vi "Queues vs Local Variables.vi"() -> ()   [LabVIEW 2011]
panel:
  in  "루프 속도(ms)":u16(ring)=50 caption="루프 속도" items=["생산자 루프와 같음"=50, "최대 속도"=0, "생산자의 2x"=25, "생산자의 1/2"=100, "생산자의 1/20"=1000]
  out "놓친 포인트 개수":i32
  in  "루프 속도(ms)":u16(ring)=50 caption="루프 속도" items=["생산자 루프와 같음"=50, "최대 속도"=0, "생산자의 2x"=25, "생산자의 1/2"=100, "생산자의 1/20"=1000]
  out "큐의 원소 개수":i32(slide) scale=0.0..1000.0
  out "생산자 루프가 \n생성한 포인트 개수":i32 caption="생산자 루프가 생성한 포인트 개수"
  in  "정지":bool
  out "로컬 변수 소비자 루프":dbl(graph) caption="사인"
  out "큐 소비자 루프":dbl(graph)=-9.510565162951542 caption="사인"
  out "생산자 루프":dbl(graph) caption="사인"
  # "생산자 루프"
  # "루프 시간 = 50 ms"
  # "로컬 변수 소비자 루프"
  # "큐 소비자 루프"
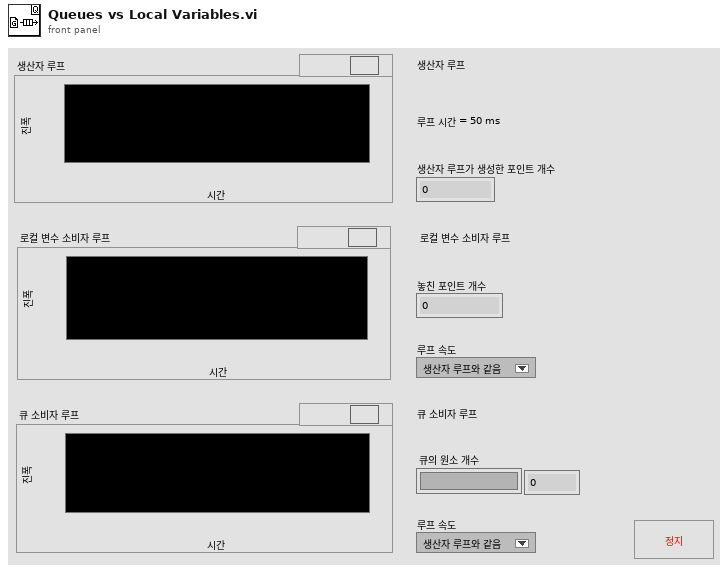
[diagram p1: front panel]
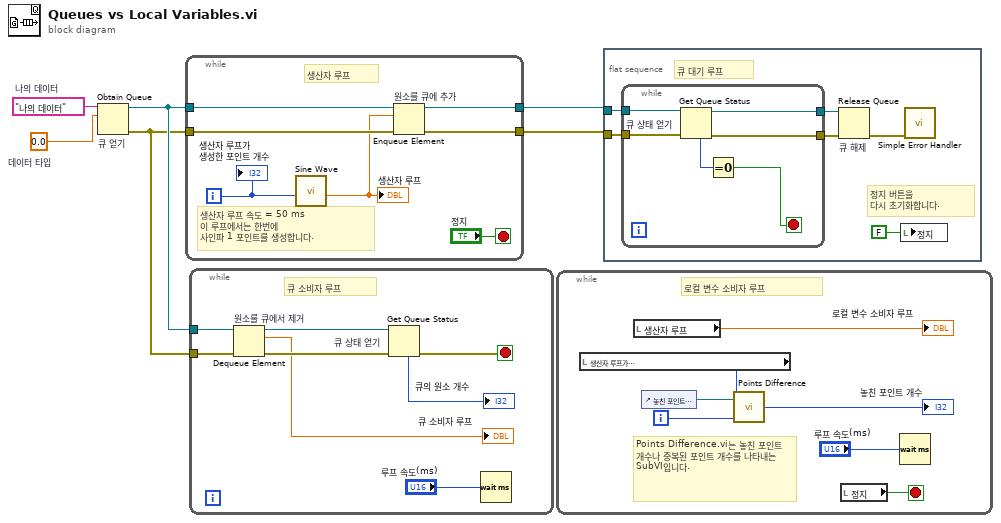
[diagram p0: block diagram]
diagram:
  w5 = "나의 데이터"  # 나의 데이터
  w6 = 0.0  # 데이터 타입
  n1 = Obtain Queue "큐 얻기"(name (unnamed)=w5, element data type=w6) -> (queue out=w4:refnum<queue>, error out=w2:errorcluster)  [unwired: 3 in, 1 out]
  n2 = while {
    tunnel: w4 -> [w11]
    tunnel: w2 -> [w10]
    tunnel: [w8] -> w1
    tunnel: [w7] -> w3
    i -> [w12]
    stop <- "정지" stop-if-true
    # "생산자 루프"
    # "생산자 루프 속도 = 50 ms\n이 루프에서는 한번에 \n사인파 1 포인트를 생성합니다."
    n3 = call "Sine Wave.vi"("숫자형"=w12) -> ("사인파"=w9:dbl)  [unwired: 6 out]
    "생산자 루프" <- w9
    n4 = Enqueue Element "원소를 큐에 추가"(queue=w11, element=w9, error in (no error)=w10) -> (queue out=w7:refnum<queue>, error out=w8:errorcluster)  [unwired: 2 out]
    "생산자 루프가 \n생성한 포인트 개수" <- w12
  }
  n5 = while {
    tunnel: w4 -> [w18]
    tunnel: w2 -> [w17]
    stop <- w15 stop-if-true
    # "큐 소비자 루프"
    n6 = Dequeue Element "원소를 큐에서 제거"(queue=w18, error in (no error)=w17) -> (queue out=w20:refnum<queue>, element=→"큐 소비자 루프":dbl, error out=w19:errorcluster)  [unwired: 2 out]
    n7 = Get Queue Status "큐 상태 얻기"(queue=w20, error in (no error)=w19) -> (error out=w15:errorcluster, # elements in queue=→"큐의 원소 개수":i32)  [unwired: 1 in, 6 out]
    n8 = Wait (ms)(milliseconds to wait="루프 속도(ms)") -> ()  [unwired: 1 out]
  }
  n9 = while {
    i -> [w26]
    stop <- w22 stop-if-true
    # "로컬 변수 소비자 루프"
    # "Points Difference.vi는 놓친 포인트 개수나 중복된 포인트 개수를 나타내는 SubVI입니다."
    n10 = local read "생산자 루프가 \n생성한 포인트 개수"() -> (w27:i32)
    n11 = local read "생산자 루프"() -> (→"로컬 변수 소비자 루프":dbl)
    n12 = control-ref of="놓친 포인트 개수"() -> (w23:refnum<vi>)
    n13 = call "Points Difference.vi"("포인트 개수(소비자 루프)"=w26, "놓친 포인트 컨트롤 참조 번호"=w23, "포인트 개수(생산자 루프)"=w27) -> ("놓친 포인트"=→"놓친 포인트 개수":i32)
    n14 = local read "정지"() -> (w22:bool)
    n15 = Wait (ms)(milliseconds to wait="루프 속도(ms)") -> ()  [unwired: 1 out]
  }
  n16 = flat-sequence {
    tunnel: w1 -> [w31]
    tunnel: w3 -> [w32]
    frame #0 {
      # "큐 대기 루프"
      # "정지 버튼을\n다시 초기화합니다."
      n17 = while {
        tunnel: w32 -> [w40]
        tunnel: w31 -> [w39]
        tunnel: [w38] -> w30
        tunnel: [w37] -> w29
        stop <- w35 stop-if-true
        n18 = Get Queue Status "큐 상태 얻기"(queue=w40, error in (no error)=w39) -> (queue out=w37:refnum<queue>, error out=w38:errorcluster, # elements in queue=w36:i32)  [unwired: 6 out]
        n19 = Equal To 0?(x=w36) -> (x = 0?=w35:bool)
      }
      n20 = Release Queue "큐 해제"(queue=w29, error in (no error)=w30) -> (error out=w33:errorcluster)  [unwired: 3 out]
      n21 = local write "정지"(FALSE ("stop")) -> ()
      n22 = call <vilib>:"Simple Error Handler.vi"("error in (no error)"=w33) -> ()  [unwired: 2 in, 7 out]
    }
  }
